vi "Fpga-6592-Top-Level.vi"() -> ()   [LabVIEW 2017]
uses:
  <vilib>/Platform/TimedLoop/XDataNode/timing_clust.ctl
  <vilib>/Platform/TimedLoop/XDataNode/nitl_modes.ctl
  <vilib>/Platform/TimedLoop/XDataNode/wakeup.ctl
  <vilib>/rvi/Emulation/niFpgaSctlEmulationGetInTimedLoop.vi
  <vilib>/rvi/Emulation/niFpgaEmulationReportErrorSimple.vi
  <vilib>/rvi/Emulation/niFpgaGetClockAttributes.vi
  <vilib>/rvi/Emulation/niFpgaCriticalErrorInLSC.vi
  <vilib>/rvi/eio/common/nirviEmuTemplateMethod_errors.vi
  <vilib>/rvi/interface/RandomDataEmulation/niFpgaRandomDataHandleErrors.vi
  <vilib>/Platform/TimedLoop/XDataNode/XDataNode.xnode
  <vilib>/eio/EIONode/EIONode.xnode
  <vilib>/rvi/DataTransferAndStorage/Container/XNode/niFpgaContainer.xnode
  <vilib>/rvi/interface/RandomDataEmulation/nirviRandomDataFpgaReadWriteTemplate.vi
  <vilib>/Platform/TimedLoop/XDataNode/XDNodeRunTimeDep.lvlib
panel:
  in  "d_mcs_i\\INTC_Interrupt":fxp<+,4,4>
  out "d_mcs_i\\gpio3_rtl_tri_o":u32
  in  "Write Interrupt":bool
  out "d_mcs_i\\gpio2_rtl_tri_o":u32
  out "d_mcs_i\\gpio_rtl_tri_o":u32
  in  "d_mcs_i\\gpio_rtl_tri_i":u32
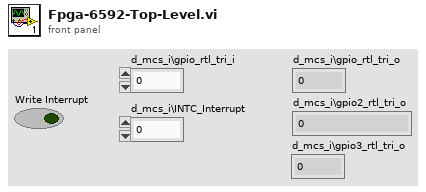
[diagram p1: front panel]
types:
  T1 = typedef "XDNodeRunTimeDep.lvlib/timing_clust.ctl" = cluster{"Expected End [f-1]":u64, "Actual End [f-1]":u64, "Finished Late? [f-1]":bool, "Expected End [i-1]":u64, "Actual End [i-1]":u64, "Finished Late? [i-1]":bool, "Expected Start [i]":u64, "Actual Start [i]":u64, "Expected Start [f]":u64, "Actual Start [f]":u64, "Source Name":string, "Structure Name":string, "Period":i64, "Deadline":i64, "Offset":i64, "Start":i64, "Priority":i32, "Timeout":i32, "Mode":T2, "Wakeup Reason":T3, "Error":errorcluster, "Source Type":string, "Secondary Source Type":string, "Global End Time":u64, "Global Start Time":u64, "Frame Duration":u64, "Iteration Duration":u64, "Assigned CPU":i32, "I/O Scan Engine Mode":u32}
  T2 = typedef "XDNodeRunTimeDep.lvlib/nitl_modes.ctl" = enum32{"No Change", "Process missed periods, maintain original phase", "Discard missed periods, maintain original phase", "Process missed periods, ignore original phase", "Discard missed periods, ignore original phase"}
  T3 = typedef "XDNodeRunTimeDep.lvlib/wakeup.ctl" = enum32{"Normal", "Aborted", "Asynchronous wakeup", "Timing source error", "Timed loop error", "Timeout"}
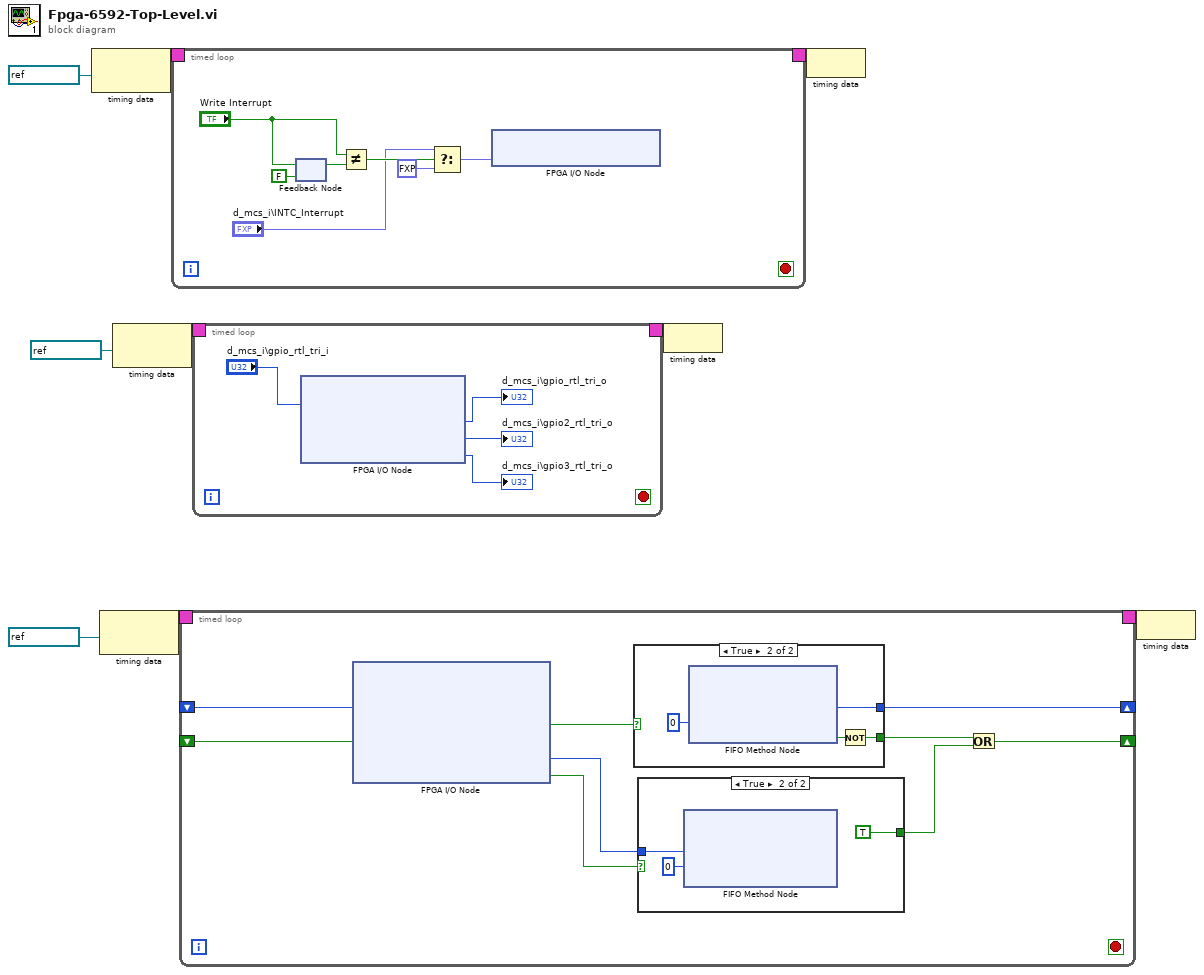
[diagram p0: block diagram]
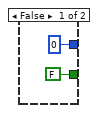
[diagram p2: hidden frame]
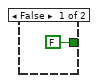
[diagram p3: hidden frame]
diagram:
  n1 = node-c288(refnum<k21> "100MHz" ("Source Name")) -> (w3:T1)
  n2 = node-c288(refnum<k21> "100MHz" ("Source Name")) -> (w9:T1)
  n3 = node-c288(refnum<k21> "100MHz" ("Source Name")) -> (w6:T1)
  n4 = timed-loop {
    timing: w3 -> [_]
    timing-out: [_] -> w2
    stop <- _ stop-if-true
    n5 = feedback-in #1("Write Interrupt") -> ()
    n6 = feedback #1(FALSE ("Write Interrupt")) -> (w16:bool)
    n7 = Not Equal?(x="Write Interrupt", y=w16) -> (x != y?=w13:bool)
    n8 = Select(t="d_mcs_i\\INTC_Interrupt", s=w13, f=fxp<+,4,4> 0.0) -> (s? t:f=w11:fxp<+,4,4>)
    n9 = xnode "FPGA I/O Node"("d_mcs_i\\INTC_Interrupt"=w11) -> ()  [unwired: 1 in, 1 out]
  }
  n10 = timed-loop {
    timing: w9 -> [_]
    timing-out: [_] -> w8
    shift-right: [w24] -> _
    shift-left: _ -> [w23]
    shift-right: [w20] -> _
    shift-left: _ -> [w19]
    stop <- _ stop-if-true
    n11 = xnode "FPGA I/O Node"("d_mcs_i\\IO_BUS_read_data"=w19, "d_mcs_i\\IO_BUS_ready"=w23) -> ("d_mcs_i\\IO_BUS_read_strobe"=w22:bool, "d_mcs_i\\IO_BUS_write_data"=w26:u32, "d_mcs_i\\IO_BUS_write_strobe"=w27:bool)  [unwired: 6 in, 7 out]
    n12 = case shown="True" w22 {
      tunnel: [FALSE w30] -> w21
      tunnel: [u32 0 ("Element") w31] -> w20
      frame False {
      }
      frame True {
        n13 = xnode ("FIFO Method Node")("Timeout"=0) -> ("Element"=w31:u32, "Timed Out?"=w32:bool)  [unwired: 1 in, 1 out]
        n14 = Not(x=w32) -> (.not. x?=w30:bool)
      }
    }
    n15 = case shown="True" w27 {
      tunnel: w26 -> [_ w36]
      tunnel: [FALSE TRUE] -> w25
      frame False {
      }
      frame True {
        n16 = xnode ("FIFO Method Node")("Element"=w36, "Timeout"=0) -> ()  [unwired: 1 in, 2 out]
      }
    }
    n17 = Or(x=w21, y=w25) -> (x .or. y?=w24:bool)
  }
  n18 = timed-loop {
    timing: w6 -> [_]
    timing-out: [_] -> w5
    stop <- _ stop-if-true
    n19 = xnode "FPGA I/O Node"("d_mcs_i\\gpio1_rtl_tri_i"="d_mcs_i\\gpio_rtl_tri_i") -> ("d_mcs_i\\gpio1_rtl_tri_o"=→"d_mcs_i\\gpio_rtl_tri_o":u32, "d_mcs_i\\gpio2_rtl_tri_o"=→"d_mcs_i\\gpio2_rtl_tri_o":u32, "d_mcs_i\\gpio3_rtl_tri_o"=→"d_mcs_i\\gpio3_rtl_tri_o":u32)  [unwired: 4 in, 4 out]
  }
  n20 = node-c288(w5) -> ()
  n21 = node-c288(w2) -> ()
  n22 = node-c288(w8) -> ()
